vi "configREF_phi.vi"(8 "error in (no error)":errorcluster, 9 "Phase (°)":dbl, 10 "REF Channel":T1=1 min=1 max=16, 11 "Instrument.Lockin in":refnum<class "Instrument.Lockin.lvclass">) -> (0 "error out":errorcluster, 3 "Instrument.Lockin out":refnum<class "Instrument.Lockin.lvclass">)   [LabVIEW 2016, in "Instrument.Lockin.lvclass"]
doc: "API to configure a REF phase.\n\nSpecify which channel you want to change and the value you want to set.\n\nIf address=\"\", this API reads from localhost\nIf address is remote lockin, you need to add this computer to allowed whitelist on the lockin computer you are trying to access."
uses:
  Instrument.Lockin.lvclass
  LockinDAQ/Typedefs/REF_Channel-Numeric.ctl
  LockinDAQ/Typedefs/Instrument.Lockin.Commands--Enum.ctl
  LockinDAQ/LockinDAQ.lvclass
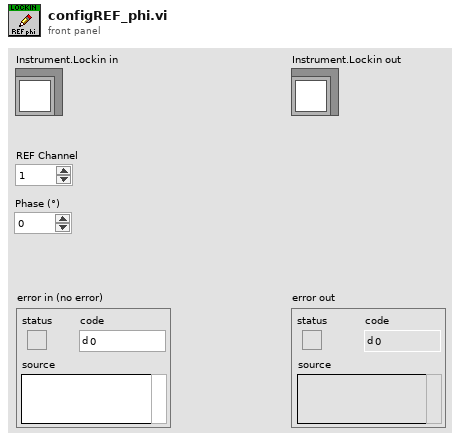
[diagram p1: front panel]
types:
  T1 = typedef "LockinDAQ.lvclass/REF_Channel-Numeric.ctl" = i32
  T2 = typedef "LockinDAQ.lvclass/Instrument.Lockin.Commands--Enum.ctl" = enum16{"configAO", "configAO_Amplitude", "configAO_DC", "configAO_Frequency", "configAO_Phase", "configAO_Function", "configAO_I+", "configREF", "configREF_Frequency", "configREF_Phase", "configREF_Filter", "configIVmode", "Reset", "configSampling", "Trigger", "getAO", "getAI", "getResults", "getTrigger", "getIVmode", "getSampling", "getAOconfig", "getREFconfig", "getREF_Filter", "configGain", "getGain", "configAutoSampling", "getAutoSampling"}
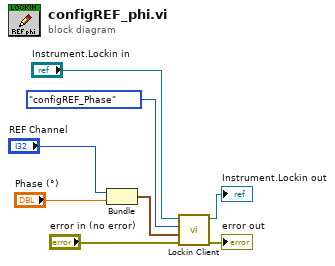
[diagram p0: block diagram]
diagram:
  n1 = Bundle("REF Channel"="REF Channel", "Phase (°)"="Phase (°)") -> (w8:cluster{"REF Channel":T1, "Phase (°)":dbl})  [unwired: 1 in]
  n2 = call "Lockin Client.vi"("error in (no error)"="error in (no error)", "Data"=w8, "Command"=Instrument.Lockin.Commands--Enum."configREF_Phase", "Instrument.Lockin in"="Instrument.Lockin in") -> ("error out"=→"error out":errorcluster, "Instrument.Lockin out"=→"Instrument.Lockin out":refnum<class "Instrument.Lockin.lvclass">)  [unwired: 5 in, 1 out]
